vi "OAT State Machine Generate Event for Boolean.vi"(1 "Initialize":bool, 2 "Boolean":bool, 4 "Action":T1(ring)) -> (7 "Event":bool)   [LabVIEW 2017]
doc: "Detects events for the boolean objects. The event of boolean range from true, false,true to false, false to true and boolean crossing. When the event detected, the coresponding output boolean is TRUE."
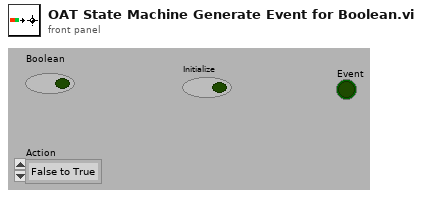
[diagram p1: front panel]
types:
  T1 = enum16{"False to True", "True to False", "Either Crossing", "True", "False"}
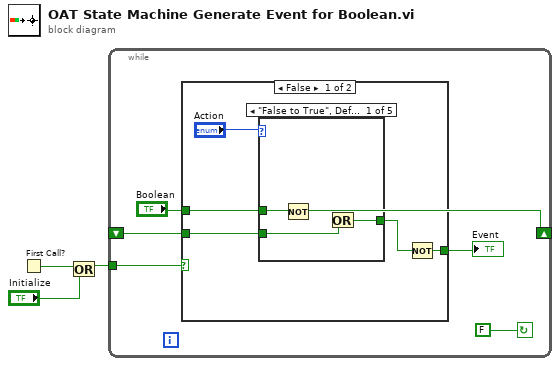
[diagram p0: block diagram]
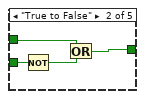
[diagram p2: hidden frame]
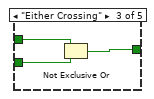
[diagram p3: hidden frame]
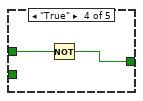
[diagram p4: hidden frame]
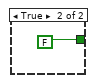
[diagram p6: hidden frame]
diagram:
  n1 = First Call?() -> (First Call?: T/F=w3:bool)
  n2 = Or(x=w3, y="Initialize") -> (x .or. y?=w2:bool)
  n3 = while {
    tunnel: w2 -> [w6]
    shift-left: _ -> [w8]
    shift-right: ["Boolean"] -> _
    stop <- FALSE continue-if-true
    n4 = case shown="False" w6 {
      tunnel: w8 -> [w13 _]
      tunnel: [w11 FALSE] -> w4
      tunnel: "Boolean" -> [w9 _]
      frame False {
        n5 = case shown="\"False to True\", Default" "Action" {
          tunnel: w9 -> [w17 w19 w24 w26 w27]
          tunnel: w13 -> [w15 w21 w23 _ _]
          tunnel: [w14 w18 w22 w25 w27] -> w12
          frame "False to True", Default {
            n6 = Not(x=w17) -> (.not. x?=w16:bool)
            n7 = Or(x=w16, y=w15) -> (x .or. y?=w14:bool)
          }
          frame "True to False" {
            n8 = Not(x=w21) -> (.not. x?=w20:bool)
            n9 = Or(x=w19, y=w20) -> (x .or. y?=w18:bool)
          }
          frame "Either Crossing" {
            n10 = Not Exclusive Or(1:w23, 2:w24) -> (0:w22:bool)
          }
          frame "True" {
            n11 = Not(x=w26) -> (.not. x?=w25:bool)
          }
          frame "False" {
          }
        }
        n12 = Not(x=w12) -> (.not. x?=w11:bool)
      }
      frame True {
      }
    }
    "Event" <- w4
  }
